vi "Create_File.vi"(8 "error in (no error)":errorcluster, 9 "Setup":string, 10 "Path":path=path "C:/Users/YuanYuan/Desktop/Labview Data/Chirp", 11 "ChirpEIS in":refnum<class "ChirpEIS.lvclass">) -> (0 "error out":errorcluster, 3 "ChirpEIS out":refnum<class "ChirpEIS.lvclass">)   [LabVIEW 2014, in "ChirpEIS.lvclass"]
uses:
  ChirpEIS.lvclass
  ChirpEIS.lvclass/ChirpEIS.ctl
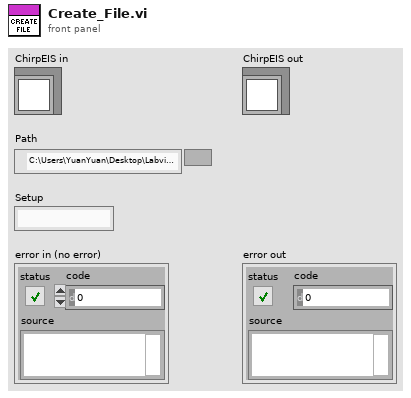
[diagram p1: front panel]
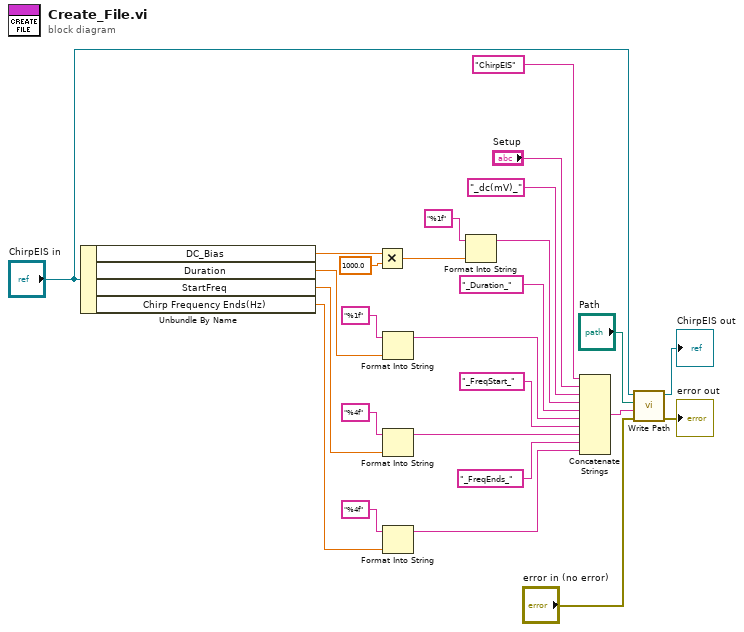
[diagram p0: block diagram]
diagram:
  n1 = Unbundle By Name("ChirpEIS in") -> ("DC_Bias"=w18:dbl, "Duration"=w11:dbl, "StartFreq"=w7:dbl, "Chirp Frequency Ends(Hz)"=w3:dbl)
  n2 = Multiply(x=w18, y=1000.0) -> (x*y=w16:dbl)
  n3 = Format Into String(format string="%1f", w11) -> (resulting string=w10:string)  [unwired: 2 in, 1 out]
  n4 = Format Into String(format string="%4f", w7) -> (resulting string=w6:string)  [unwired: 2 in, 1 out]
  n5 = Format Into String(format string="%4f", w3) -> (resulting string=w2:string)  [unwired: 2 in, 1 out]
  n6 = Format Into String(format string="%1f", w16) -> (resulting string=w20:string)  [unwired: 2 in, 1 out]
  n7 = Concatenate Strings("ChirpEIS" ("name or relative path"), "Setup", "_dc(mV)_" ("name or relative path"), w20, "_Duration_" ("name or relative path"), w10, "_FreqStart_" ("name or relative path"), w6, "_FreqEnds_" ("name or relative path"), w2) -> (w24:string)
  n8 = call "Write Path.vi"("error in (no error)"="error in (no error)", "Experiment name"=w24, "Path"="Path", "ChirpEIS In"="ChirpEIS in") -> ("error out"=→"error out":errorcluster, "ChirpEIS out"=→"ChirpEIS out":refnum<class "ChirpEIS.lvclass">)  [unwired: 6 in]
